vi "delayed_replace_star.vi"() -> ()   [LabVIEW 2010, in "password.xctl"]
uses:
  password.xctl
  controls/Data.ctl
panel:
  in  "delay":u32=1000 caption="delay (1000)"
  in  "display ref":refnum<vi>
  in  "new val":T1
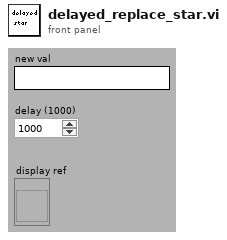
[diagram p1: front panel]
types:
  T1 = typedef "password.xctl/Data.ctl" = string
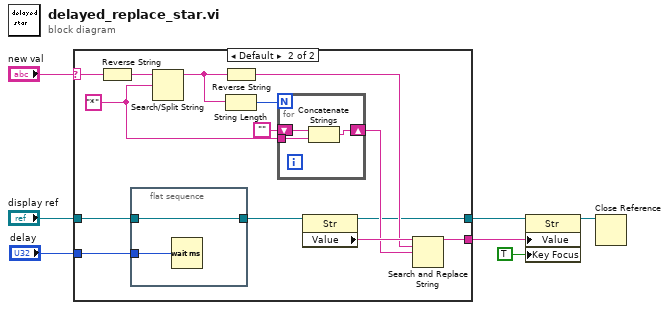
[diagram p0: block diagram]
diagram:
  n1 = case shown="Default" "new val" {
    selector: "new val" -> [_ w12]
    tunnel: "display ref" -> [w8 w14]
    tunnel: "delay" -> [_ w11]
    tunnel: [w8 w10] -> w3
    tunnel: [_ w9] -> w2
    frame "\u0000" {
    }
    frame Default {
      w22 = "*"
      n2 = Reverse String(1:w12) -> (0:w19:string)
      n3 = flat-sequence {
        tunnel: w14 -> [w24]
        tunnel: [w24] -> w13
        tunnel: w11 -> [w23]
        frame #0 {
          n4 = Wait (ms)(milliseconds to wait=w23) -> ()  [unwired: 1 out]
        }
      }
      n5 = Search/Split String(string=w19, search string/char (-)=w22) -> (substring before match=w20:string)  [unwired: 1 in, 2 out]
      n6 = Reverse String(1:w20) -> (0:w16:string)
      n7 = String Length(string=w20) -> (length=w18:i32)
      n8 = for {
        N: w18 -> [_]
        shift-right: [w26] -> w15
        shift-left: "" -> [w27]
        tunnel: w22 -> [w25]
        n9 = Concatenate Strings(w27, w25) -> (w26:string)
      }
      n10 = property class="Str"(reference=w13) -> (reference out=w10:refnum<vi>, "Value"=w17:string)  [unwired: 1 in, 1 out]
      n11 = Search and Replace String(input string=w17, search string=w16, replace string=w15) -> (result string=w9:string)  [unwired: 5 in, 3 out]
    }
  }
  n12 = property class="Str"(reference=w3, "Value"=w2, "Key Focus"=TRUE) -> (reference out=w1:refnum<vi>)  [unwired: 1 in, 1 out]
  n13 = Close Reference(reference=w1) -> ()  [unwired: 1 in, 1 out]
